vi "Continuous Triggered Acquisition.vi"() -> ()   [LabVIEW 2021]
doc: "Use this VI as a template to design an application that acquires multiple records of data from the NI PXIe-5170R/5171R."
uses:
  <instrlib>/_niInstr/Multirecord Acquisition/Interface/v1/Host/Public/Requested Record Info.ctl
  <instrlib>/_niInstr/Multirecord Acquisition/Interface/v1/Host/Public/Full Record Status.ctl
  <instrlib>/_niInstr/Multirecord Acquisition/Interface/v1/Host/Public/Record State.ctl
  <instrlib>/_niInstr/Multirecord Acquisition/Interface/v1/Host/Public/Record Status.ctl
  <instrlib>/_niInstr/Data Trigger/v1/Shared/Public/Level Configuration Trigger When.ctl
  <vilib>/FPGAPlugInAG/PXIe-5170R (8CH)/niLvFpga_Open_PXIe-5170R (8CH).vi
  <vilib>/rvi/interface/common/dynamic/niFpgaDynamicAddResources.vi
  <vilib>/FPGAPlugInAG/Dynamic/niLvFpga_Close_Dynamic.vi
  <vilib>/rvi/interface/nirviOpenFPGA/nirviOpenFPGA.xnode
  FPGA Bitfiles/Multirecord_Acquisition_NI_PXIe-5170R_8CH.lvbitx
  <vilib>/rvi/interface/nirviCloseFPGA/nirviCloseFPGA.xnode
  Device Session/Device Session.lvclass
  <instrlib>/_niInstr/Data Trigger/v1/Shared/niInstr Data Trigger v1 Shared.lvlib
  <instrlib>/_niInstr/Multirecord Acquisition/Interface/v1/Host/niInstr Multirecord Acquisition v1 Host.lvclass
panel:
  out "requested records info 2":T1[](array[typedef])
  out "Waveform Graph Channel 1":T2(graph)
  out "records done 2":u64
  out "overflow occurred":bool
  out "overflow occurred 2":bool
  out "current record status 2":T3
  out "record status 2":T4
  in  "record number 2":u64
  in  "Stop":bool
  out "current record status":T3
  out "records done":u64
  out "record status":T4
  in  "pretrigger samples":u64=100
  in  "record number":u64
  out "Waveform Graph Channel 0":T2(graph)
  in  "number of samples":u64=5000
  in  "channels to configure":string="0,1"
  out "error out":errorcluster
  out "requested records info":T1[](array[typedef])
  in  "RIO Device":tag="5170"
  # "RIO Device"
  # "Channels"
  # "Acquisition Settings"
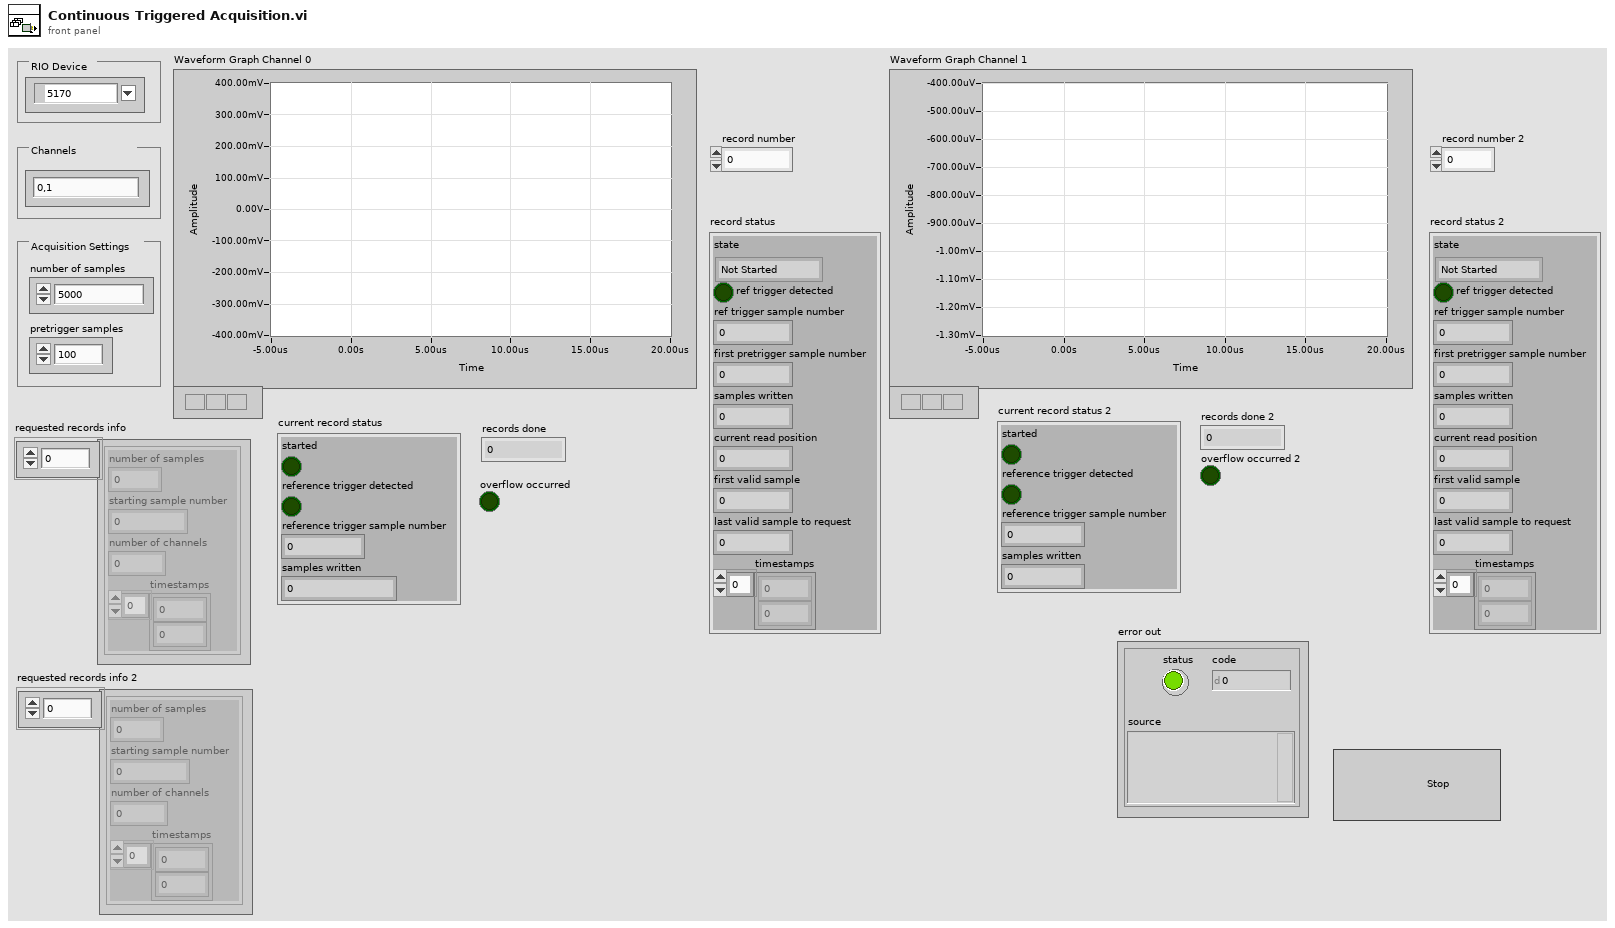
[diagram p1: front panel]
types:
  T1 = typedef "niInstr Multirecord Acquisition v1 Host.lvclass/Requested Record Info.ctl" = cluster{"number of samples":u64, "starting sample number":u64, "number of channels":u64, "timestamps":u64[]}
  T2 = cluster{"relativeX":dbl, "sample rate":dbl, "data in":dbl[]}[]
  T3 = typedef "niInstr Multirecord Acquisition v1 Host.lvclass/Record Status.ctl" = cluster{"started":bool, "reference trigger detected":bool, "reference trigger sample number":u64, "samples written":u64}
  T4 = typedef "niInstr Multirecord Acquisition v1 Host.lvclass/Full Record Status.ctl" = cluster{"state":T5, "ref trigger detected":bool, "ref trigger sample number":u64, "first pretrigger sample number":u64, "samples written":u64, "current read position":u64, "first valid sample":u64, "last valid sample to request":u64, "timestamps":u64[]}
  T5 = typedef "niInstr Multirecord Acquisition v1 Host.lvclass/Record State.ctl" = enum16{"Not Started", "Being Acquired", "Completed", "Overwritten"}
  T6 = typedef "niInstr Data Trigger v1 Shared.lvlib/Level Configuration Trigger When.ctl" = enum8{"Trigger Above", "Trigger Below"}
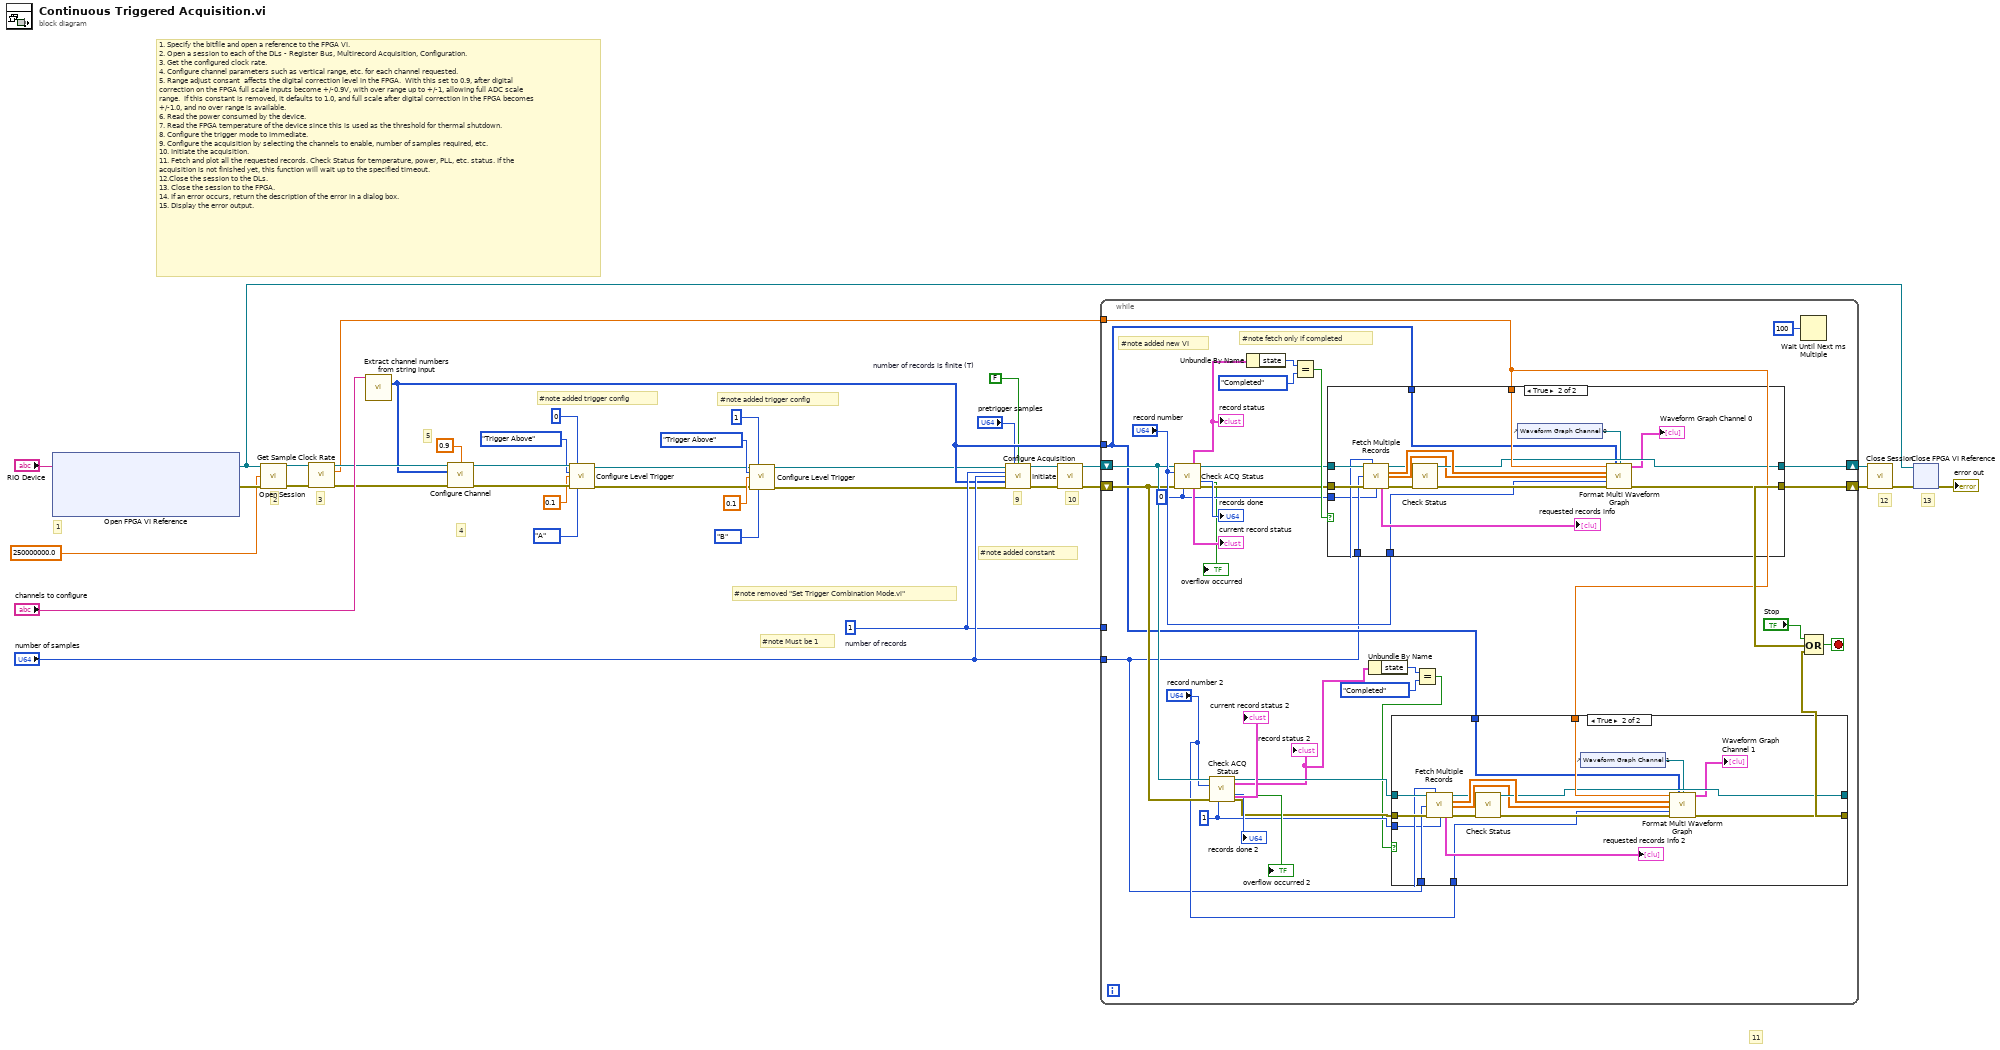
[diagram p0: block diagram]
diagram:
  w16 = 250000000.0 items=["250 MHz"=250000000.0, "200 MHz"=200000000.0, "150 MHz"=150000000.0] ("onboard sample clock rate")
  w19 = u64 1  # number of records
  w9 = FALSE  # number of records is finite (T)
  # "#note removed \"Set Trigger Combination Mode.vi\""
  # "#note added trigger config"
  # "#note Must be 1"
  # "#note added constant"
  # "#note added trigger config"
  # "5"
  # "13"
  # "12"
  # "11"
  # "10"
  # "9"
  # "4"
  # "3"
  # "1"
  # "2"
  # "1. Specify the bitfile and open a reference to the FPGA VI.\n2. Open a session to each of the DLs - Register Bus, Multirecord Acquisition, Configuration.\n3. Get the configured clock rate.\n4. Configure channel parameters such as vertical range, etc. for each channel requested.\n5. Range adjust consant  affects the digital correction level in the FPGA.  With this set to 0.9, after digital correction on the FPGA full scale inputs become +/-0.9V, with over range up to +/-1, allowing full ADC scale range.  If this constant is removed, it defaults to 1.0, and full scale after digital correction in the FPGA becomes +/-1.0, and no over range is available.\n6. Read the power consumed by the device.\n7. Read the FPGA temperature of the device since this is used as the threshold for thermal shutdown.\n8. Configure the trigger mode to Immediate.\n9. Configure the acquisition by selecting the channels to enable, number of samples required, etc.\n10. Initiate the acquisition.\n11. Fetch and plot all the requested records. Check Status for temperature, power, PLL, etc. status. If the acquisition is not finished yet, this function will wait up to the specified timeout.\n12.Close the session to the DLs.\n13. Close the session to the FPGA.\n14. If an error occurs, return the description of the error in a dialog box.\n15. Display the error output."
  n1 = xnode "Open FPGA VI Reference"("resource name"="RIO Device") -> ("FPGA VI Reference Out"=w23:refnum<k20>, "error out"=w24:errorcluster)  [unwired: 1 in]
  n2 = call "Open Session.vi"("fpga reference in"=w23, "adc clock rate (Hz)"=w16, "error in"=w24) -> ("device session out"=w28:refnum<class "Device Session.lvclass">, "error out"=w29:errorcluster)  [unwired: 11 in]
  n3 = call "Get Sample Clock Rate.vi"("device session in"=w28, "error in"=w29) -> ("device session out"=w27:refnum<class "Device Session.lvclass">, "sample clock rate (Hz)"=w18:dbl, "error out"=w26:errorcluster)  [unwired: 11 in]
  n4 = call "Extract channel numbers from string input.vi"("channel input"="channels to configure") -> ("array of chans"=w15:u32[])  [unwired: 13 in, 1 out]
  n5 = call "Configure Channel.vi"("device session in"=w27, "range adjust"=0.9, "channels"=w15, "error in"=w26) -> ("device session out"=w21:refnum<class "Device Session.lvclass">, "error out"=w20:errorcluster)  [unwired: 10 in]
  n6 = call "Configure Level Trigger.vi"("device session in"=w21, "trigger source"=u8 0, "trigger when"=Level_Configuration_Trigger_When."Trigger Above", "trigger level (V)"=0.1, "error in"=w20, "instance"=enum16{"A", "B"}."A") -> ("device session out"=w3:refnum<class "Device Session.lvclass">, "error out"=w4:errorcluster)  [unwired: 8 in]
  n7 = call "Configure Level Trigger.vi"("device session in"=w3, "trigger source"=u8 1, "trigger when"=Level_Configuration_Trigger_When."Trigger Above", "trigger level (V)"=0.1, "error in"=w4, "instance"=enum16{"A", "B"}."B") -> ("device session out"=w2:refnum<class "Device Session.lvclass">, "error out"=w1:errorcluster)  [unwired: 8 in]
  n8 = call "Configure Acquisition.vi"("device session in"=w2, "pretrigger samples"="pretrigger samples", "number of records is finite (T)"=w9, "number of records"=w19, "number of samples"="number of samples", "channels to store"=w15, "error in"=w1) -> ("device session out"=w38:refnum<class "Device Session.lvclass">, "error out"=w37:errorcluster)  [unwired: 6 in, 1 out]
  n9 = call "Initiate.vi"("device session in"=w38, "error in"=w37) -> ("device session out"=w35:refnum<class "Device Session.lvclass">, "error out"=w36:errorcluster)  [unwired: 12 in]
  n10 = while {
    tunnel: "number of samples" -> [w44]
    tunnel: w18 -> [w43]
    shift-right: [w69] -> w30
    shift-left: w36 -> [w55]
    shift-right: [w71] -> w31
    shift-left: w35 -> [w56]
    tunnel: w15 -> [w47]
    tunnel: w19 -> [_]
    stop <- w70 stop-if-true
    w50 = u8 1 ("channel")
    w57 = u8 0 ("channel")
    # "#note fetch only if completed"
    # "#note added new VI"
    n11 = call "Check ACQ Status.vi"("device session in"=w56, "record number"="record number", "error in"=w55, "channel"=w57) -> ("record status"=w66:T4, "device session out"=w60:refnum<class "Device Session.lvclass">, "records done"=→"records done":u64, "overflow occurred"=→"overflow occurred":bool, "current record status"=→"current record status":T3, "error out"=w59:errorcluster)  [unwired: 6 in]
    "record status" <- w66
    n12 = call "Check ACQ Status.vi"("device session in"=w56, "record number"="record number 2", "error in"=w55, "channel"=w50) -> ("record status"=w40:T4, "device session out"=w46:refnum<class "Device Session.lvclass">, "records done"=→"records done 2":u64, "overflow occurred"=→"overflow occurred 2":bool, "current record status"=→"current record status 2":T3, "error out"=w45:errorcluster)  [unwired: 6 in]
    "record status 2" <- w40
    n13 = Unbundle By Name(w66) -> ("state"=w65:T5)
    n14 = Equal?(x=w65, y=Record_State."Completed" ("state")) -> (x = y?=w63:bool)
    n15 = case shown="True" w63 {
      tunnel: w43 -> [_ w108]
      tunnel: [w91 w106] -> w71
      tunnel: w47 -> [_ w105]
      tunnel: [w92 w100] -> w69
      tunnel: w60 -> [w91 w99]
      tunnel: w59 -> [w92 w98]
      tunnel: w44 -> [_ w97]
      tunnel: "record number" -> [_ w96]
      tunnel: w57 -> [_ w93]
      frame False {
      }
      frame True {
        n16 = call "Fetch Multiple Records.vi"("device session in"=w99, "starting record"=w96, "number of samples"=w97, "error in"=w98, "channel"=w93) -> ("device session out"=w101:refnum<class "Device Session.lvclass">, "data"=w109:dbl[][], "relativeX (samples)"=w104:dbl[], "requested records info"=→"requested records info":T1[], "error out"=w103:errorcluster)  [unwired: 6 in]
        n17 = call "Check Status.vi"("device session in"=w101, "error in"=w103) -> ("device session out"=w106:refnum<class "Device Session.lvclass">, "error out"=w102:errorcluster)  [unwired: 12 in]
        n18 = control-ref of="Waveform Graph Channel 0"() -> (w95:refnum<vi>)
        n19 = call "Format Multi Waveform Graph.vi"("sample rate (Hz)"=w108, "array of chans"=w105, "waveform graph"=w95, "data in"=w109, "relativeX (samples)"=w104, "start record number"=w96, "error in"=w102) -> ("waveform out"=→"Waveform Graph Channel 0":T2, "error out"=w100:errorcluster)  [unwired: 7 in]
      }
    }
    n20 = Unbundle By Name(w40) -> ("state"=w41:T5)
    n21 = Equal?(x=w41, y=Record_State."Completed" ("state")) -> (x = y?=w39:bool)
    n22 = case shown="True" w39 {
      tunnel: w43 -> [_ w89]
      tunnel: [w72 w87] -> _
      tunnel: w47 -> [_ w86]
      tunnel: [w73 w81] -> w48
      tunnel: w46 -> [w72 w80]
      tunnel: w45 -> [w73 w79]
      tunnel: w44 -> [_ w78]
      tunnel: "record number 2" -> [_ w77]
      tunnel: w50 -> [_ w74]
      frame False {
      }
      frame True {
        n23 = call "Fetch Multiple Records.vi"("device session in"=w80, "starting record"=w77, "number of samples"=w78, "error in"=w79, "channel"=w74) -> ("device session out"=w82:refnum<class "Device Session.lvclass">, "data"=w90:dbl[][], "relativeX (samples)"=w85:dbl[], "requested records info"=→"requested records info 2":T1[], "error out"=w84:errorcluster)  [unwired: 6 in]
        n24 = call "Check Status.vi"("device session in"=w82, "error in"=w84) -> ("device session out"=w87:refnum<class "Device Session.lvclass">, "error out"=w83:errorcluster)  [unwired: 12 in]
        n25 = control-ref of="Waveform Graph Channel 1"() -> (w76:refnum<vi>)
        n26 = call "Format Multi Waveform Graph.vi"("sample rate (Hz)"=w89, "array of chans"=w86, "waveform graph"=w76, "data in"=w90, "relativeX (samples)"=w85, "start record number"=w77, "error in"=w83) -> ("waveform out"=→"Waveform Graph Channel 1":T2, "error out"=w81:errorcluster)  [unwired: 7 in]
      }
    }
    n27 = Wait Until Next ms Multiple(millisecond multiple=u32 100) -> ()  [unwired: 1 out]
    n28 = Compound Arithmetic op=OR("Stop", w69, w48) -> (w70:bool)
  }
  n29 = call "Close Session.vi"("device session in"=w31, "error in"=w30) -> ("error out"=w22:errorcluster)  [unwired: 13 in]
  n30 = xnode "Close FPGA VI Reference"("FPGA VI Reference In"=w23, "error in"=w22) -> ("error out"=→"error out":errorcluster)
